vi "FTW-Subscriber-Construct.vi"(5 "Publisher Address":string, 7 "Receive Message Size Limit":i32=1000 format="%_4pbytes", 9 "Linger":i32=200 format="%d msec", 11 "error in":errorcluster) -> (4 "FTW Subscriber":refnum<data-value>, 6 "Subscription":refnum<event-registration>, 15 "error out":errorcluster)   [LabVIEW 2015]
uses:
  core/FTW-Subscriber-Core-Type.ctl
panel:
  # "Inputs"
  # "Outputs"
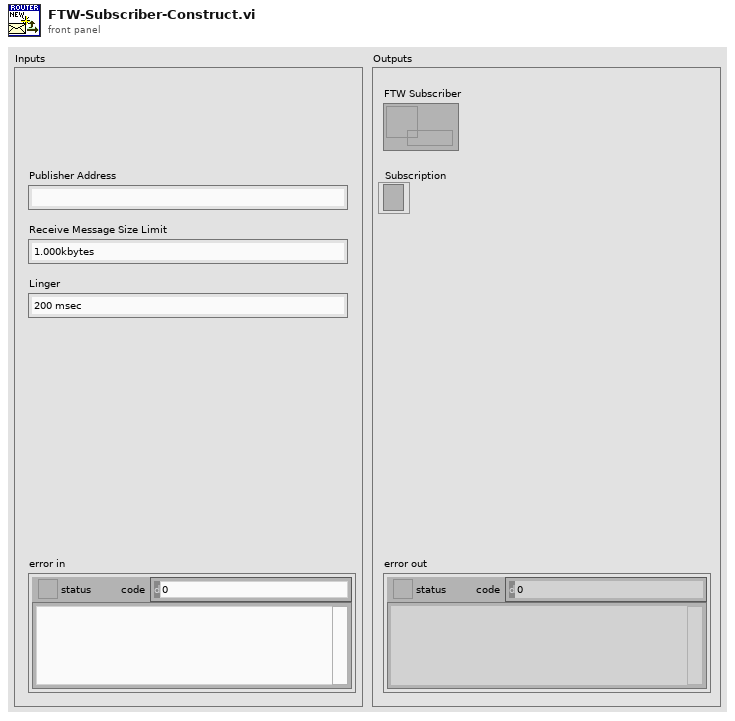
[diagram p1: front panel]
types:
  T1 = typedef "FTW-Subscriber-Core-Type.ctl" = cluster{"Socket":i64, "SubscriptionEvent":refnum<user-event>}
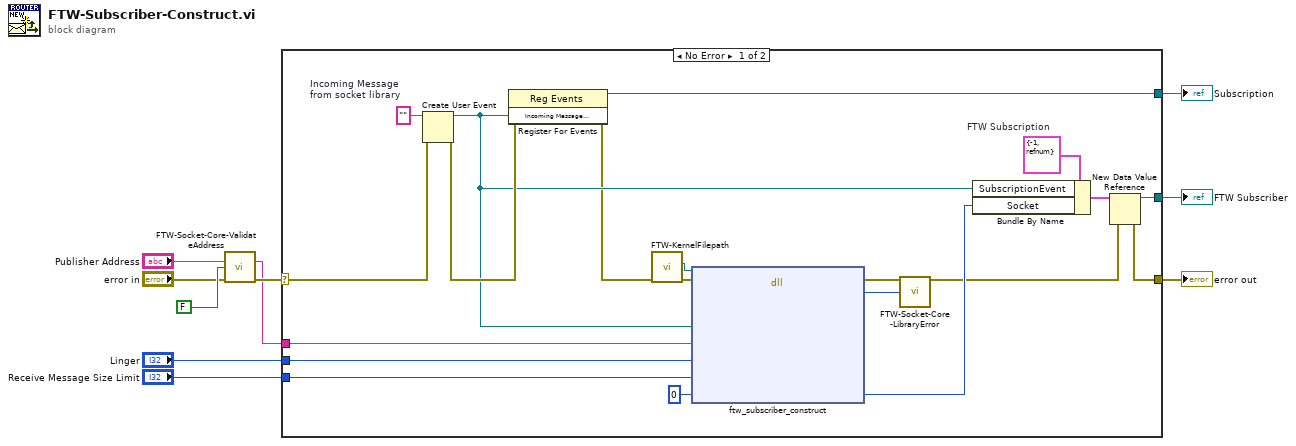
[diagram p0: block diagram]
diagram:
  n1 = call "FTW-Socket-Core-ValidateAddress.vi"("Address"="Publisher Address", "Allow wildcard replacement?"=FALSE, "error in"="error in") -> ("Sanitized Address"=w6:string, "error out"=w8:errorcluster)  [unwired: 10 in, 1 out]
  n2 = case shown="No Error" w8 {
    selector: w8 -> [w18 w31]
    tunnel: [w24 _] -> w10
    tunnel: [w22 w31] -> w9
    tunnel: [w16 _] -> w4
    tunnel: w6 -> [w29 _]
    tunnel: "Linger" -> [w21 _]
    tunnel: "Receive Message Size Limit" -> [w20 _]
    frame No Error {
      w15 = T1 {"Socket"=-1, "SubscriptionEvent"=refnum}  # FTW Subscription
      w19 = ""  # Incoming Message from socket library
      n3 = Create User Event(user event datatype=w19, error in=w18) -> (user event=w14:refnum<user-event>, error out=w17:errorcluster)
      n4 = register-events(error in=w17, w14) -> (reference out=w16:refnum<event-registration>, error out=w13:errorcluster)  [unwired: 1 in]
      n5 = call "FTW-KernelFilepath.vi"("error in"=w13) -> ("error out"=w11:errorcluster, "Library Filepath"=w12:path)  [unwired: 8 in, 1 out]
      n6 = dll-call lib="?" fn="ftw_subscriber_construct"(path in=w12, error in=w11, "Incoming Message Event"=w14, "Address"=w29, "Linger (msec)"=w21, "Max Recv Size (bytes)"=w20, "Socket Handle"=i64 0) -> (error out=w30:errorcluster, "Return Value"=w28:i64, "Socket Handle"=w26:i64)  [unwired: 7 in, 1 out]
      n7 = call "FTW-Socket-Core-LibraryError.vi"("error in"=w30, "Return Value"=w28) -> ("error out"=w23:errorcluster)  [unwired: 13 in]
      n8 = Bundle By Name(cluster=w15, "SubscriptionEvent"=w14, "Socket"=w26) -> (w25:T1)
      n9 = New Data Value Reference(data value=w25, error in=w23) -> (data value reference=w24:refnum<data-value>, error out=w22:errorcluster)
    }
    frame Error {
    }
  }
  "error out" <- w9
  "FTW Subscriber" <- w10
  "Subscription" <- w4
